vi "Controller Set and Check PS Status.vi"(7 "PS ON-OFF":u8[](array[numeric]), 8 "error in (no error)":errorcluster, 10 "PS Status Variables":refnum<k21>[](array[refnum]), 11 "PS ON-OFF Variables":refnum<k21>[](array[refnum])) -> (0 "error out":errorcluster, 2 "Status Error Matrix":bool[][](array[boolean]), 3 "No Error":bool)   [LabVIEW 2011, in "Controller VIs.lvlib"]
uses:
  Controller VIs.lvlib
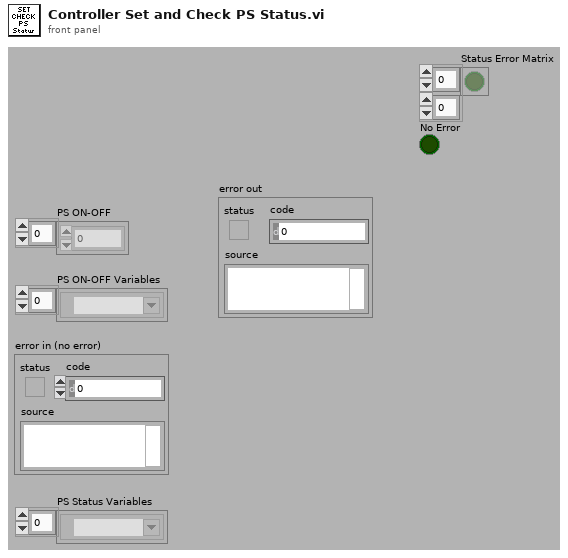
[diagram p1: front panel]
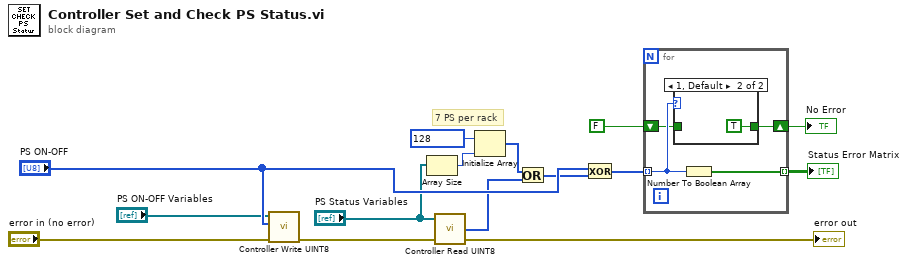
[diagram p0: block diagram]
diagram:
  # "7 PS per rack"
  n1 = call "Controller Write UINT8.vi"("error in (no error)"="error in (no error)", "Values"="PS ON-OFF", "Variables"="PS ON-OFF Variables") -> ("error out"=w6:errorcluster)  [unwired: 8 in]
  n2 = Array Size(array="PS Status Variables") -> (size(s)=w3:i32)
  n3 = call "Controller Read UINT8.vi"("error in (no error)"=w6, "Variables"="PS Status Variables") -> ("error out"=→"error out":errorcluster, "Values"=w2:u8[])  [unwired: 2 in]
  n4 = Initialize Array(u8 128, w3) -> (w1:u8[])
  n5 = Or(x=w1, y=w2) -> (x .or. y?=w8:u8[])
  n6 = Exclusive Or(1:w8, 2:"PS ON-OFF") -> (0:w13:u8[])
  n7 = for {
    tunnel: w13 -> [w18] mode=indexing
    tunnel: [w19] -> w12 mode=indexing
    shift-right: [w17] -> w10
    shift-left: FALSE -> [w16]
    n8 = case shown="1, Default" w18 {
      tunnel: [w20 TRUE] -> w17
      tunnel: w16 -> [w20 _]
      frame 0 {
      }
      frame 1, Default {
      }
    }
    n9 = Number To Boolean Array(number=w18) -> (Boolean array=w19:bool[])
  }
  "Status Error Matrix" <- w12
  "No Error" <- w10
